vi "simulate camera image.vi"(8 "error in (no error)":errorcluster, 11 "FakeCamera in":refnum<class "Point Grey Camera.lvclass">) -> (0 "error out":errorcluster, 2 "Acquisition OK?":bool, 3 "FakeCamera out":refnum<class "Point Grey Camera.lvclass">, 5 "acq time (ms)":u32)   [LabVIEW 2020, in "Point Grey Camera.lvclass"]
uses:
  Point Grey Camera.lvclass
  Point Grey Camera.lvclass/Point Grey Camera.ctl
  NI_Vision_Development_Module.lvlib
panel:
  in  "dont flip":bool
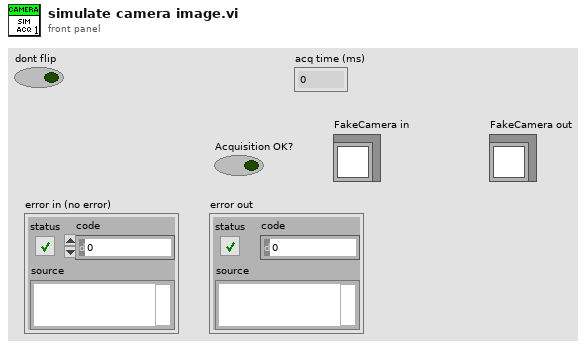
[diagram p1: front panel]
types:
  T1 = typedef "IMAQ Image.ctl" = refnum<image>
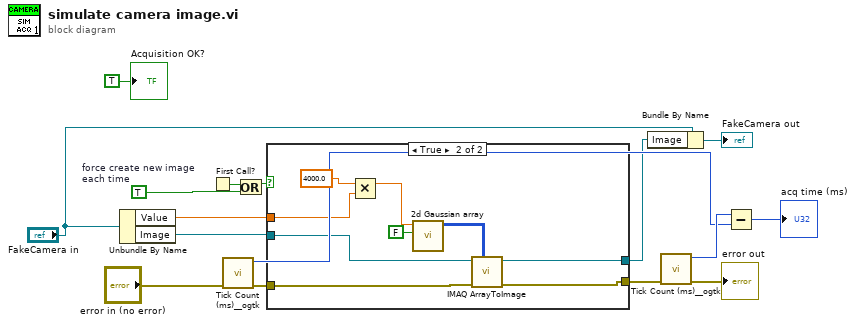
[diagram p0: block diagram]
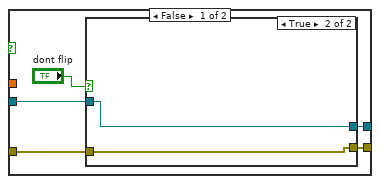
[diagram p2: hidden frame]
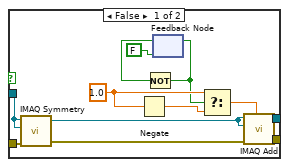
[diagram p3: hidden frame]
diagram:
  w1 = TRUE  # force create new image each time
  n1 = Unbundle By Name("FakeCamera in") -> ("Value"=w3:dbl, "Image"=w8:T1)
  n2 = First Call?() -> (First Call?: T/F=w4:bool)
  n3 = call "Tick Count (ms)__ogtk.vi"("error in (no error)"="error in (no error)") -> ("error out"=w10:errorcluster, "millisecond timer value"=w12:u32)  [unwired: 9 in]
  n4 = Or(x=w4, y=w1) -> (x .or. y?=w2:bool)
  n5 = case shown="True" w2 {
    tunnel: w10 -> [w20 w44]
    tunnel: [w18 w43] -> w15
    tunnel: [w19 w42] -> w7
    tunnel: w8 -> [w21 w41]
    tunnel: w3 -> [_ w36]
    frame False {
      n6 = case shown="True" "dont flip" {
        tunnel: w21 -> [w33 w35]
        tunnel: w20 -> [w32 w34]
        tunnel: [w24 w35] -> w19
        tunnel: [w23 w34] -> w18
        frame False {
          w28 = 1.0 ("Constant")
          n7 = call "IMAQ Symmetry"("error in (no error)"=w32, "Image Dst"=w33, "Image Src"=w33) -> ("error out"=w22:errorcluster, "Image Dst Out"=w31:T1)  [unwired: 2 in]
          n8 = Negate(x=w28) -> (-x=w27:dbl)
          n9 = feedback #1(FALSE) -> (w30:bool)
          n10 = Not(x=w30) -> (.not. x?=w26:bool)
          n11 = feedback-in #1(w26) -> ()
          n12 = Select(t=w28, s=w26, f=w27) -> (s? t:f=w25:dbl)
          n13 = call "IMAQ Add"("Image Src A"=w31, "Constant"=w25, "Image Dst"=w31, "error in (no error)"=w22) -> ("Image Dst Out"=w24:T1, "error out"=w23:errorcluster)  [unwired: 3 in]
        }
        frame True {
        }
      }
    }
    frame True {
      n14 = Multiply(x=4000.0 ("A"), y=w36) -> (x*y=w37:dbl)
      n15 = call "2d Gaussian array.vi"("multiply A by random number"=FALSE, "A"=w37) -> ("Intensity Graph"=w40:u16[][])  [unwired: 9 in]
      n16 = call "IMAQ ArrayToImage"("Image Pixels (U16)"=w40, "error in (no error)"=w44, "Image"=w41) -> ("error out"=w43:errorcluster, "Image Out"=w42:T1)  [unwired: 7 in]
    }
  }
  n17 = Bundle By Name(cluster="FakeCamera in", "Image"=w7) -> (→"FakeCamera out":refnum<class "Point Grey Camera.lvclass">)
  n18 = call "Tick Count (ms)__ogtk.vi"("error in (no error)"=w15) -> ("error out"=→"error out":errorcluster, "millisecond timer value"=w13:u32)  [unwired: 9 in]
  n19 = Subtract(x=w13, y=w12) -> (x-y=→"acq time (ms)":u32)
  "Acquisition OK?" <- TRUE ("Acquisition OK?")
